vi "Version_2.0_Single_Column_Code.vi"() -> ()   [LabVIEW 2020] (continued)
                                n401 = local read "VISA Refnum in\nfor Pump"() -> (w876:refnum<visa-resource-name>)
                                n402 = local read "Port for \nA1-Equilibriation"() -> (w875:string)
                                n403 = call "PortChanger (SubVI).vi"("Port Number"=w875, "VISA Refnum in"=w876) -> ()  [unwired: 10 in]
                                }
                                frame #1 {
                                n404 = local read "VISA Refnum in\nfor Pump"() -> (w877:refnum<visa-resource-name>)
                                n405 = call "ProcessCompletionWaiter (SubVI).vi"("VISA Refnum in"=w877) -> ()  [unwired: 11 in]
                                }
                                frame #2 {
                                n406 = local read "VISA Refnum in\nfor Pump"() -> (w882:refnum<visa-resource-name>)
                                n407 = local read "Apparent Volume\nof Syringe"() -> (w878:dbl)
                                n408 = local read "Volume of Syringe"() -> (w879:dbl)
                                n409 = call "RPickUp(SubVI).vi"("Volume to be picked up"=w878, "Volume of Syringe"=w879, "Resolution of PickUP"=T2."Standard Pumping", "PickUp Flow Rate (ul/min)"=150.0, "VISA Refnum in"=w882) -> ()  [unwired: 6 in, 1 out]
                                }
                                frame #3 {
                                n410 = local read "Stopper that ends \nthe main loops"() -> (w883:bool)
                                n411 = local read "VISA Refnum in\nfor Pump"() -> (w884:refnum<visa-resource-name>)
                                n412 = case shown="True" w883 {
                                frame False {
                                }
                                frame True {
                                n413 = local read "VISA Refnum in\nfor Pump"() -> (w885:refnum<visa-resource-name>)
                                n414 = call "HardStopCurrentProcess (SubVI).vi"("VISA Refnum in"=w885) -> ()  [unwired: 11 in]
                                }
                                }
                                n415 = call "ProcessCompletionWaiter (SubVI).vi"("VISA Refnum in"=w884) -> ()  [unwired: 11 in]
                                }
                                frame #4 {
                                n416 = local read "VISA Refnum in\nfor Pump"() -> (w887:refnum<visa-resource-name>)
                                n417 = call "PortChanger (SubVI).vi"("Port Number"="1", "VISA Refnum in"=w887) -> ()  [unwired: 10 in]
                                }
                                frame #5 {
                                n418 = local read "Stopper that ends \nthe main loops"() -> (w888:bool)
                                n419 = local read "VISA Refnum in\nfor Pump"() -> (w889:refnum<visa-resource-name>)
                                n420 = case shown="True" w888 {
                                frame False {
                                }
                                frame True {
                                n421 = local read "VISA Refnum in\nfor Pump"() -> (w890:refnum<visa-resource-name>)
                                n422 = call "HardStopCurrentProcess (SubVI).vi"("VISA Refnum in"=w890) -> ()  [unwired: 11 in]
                                }
                                }
                                n423 = call "ProcessCompletionWaiter (SubVI).vi"("VISA Refnum in"=w889) -> ()  [unwired: 11 in]
                                }
                                frame #6 {
                                n424 = local read "VISA Refnum in\nfor Pump"() -> (w895:refnum<visa-resource-name>)
                                n425 = local read "Volume of Syringe"() -> (w892:dbl)
                                n426 = call "GoToAbsolutePosition(SubVI).vi"("Absolute Volume Position in Syringe (in ul)"=0.0 ("Volume to be picked up"), "Volume of Syringe"=w892, "Resolution of Pumping"=T2."Standard Pumping" ("Resolution of PickUP"), "Flow Rate (ul/min)"=150.0 ("PickUp Flow Rate (ul/min)"), "VISA Refnum in"=w895) -> ()  [unwired: 6 in, 1 out]
                                }
                                frame #7 {
                                n427 = local read "Stopper that ends \nthe main loops"() -> (w896:bool)
                                n428 = local read "VISA Refnum in\nfor Pump"() -> (w897:refnum<visa-resource-name>)
                                n429 = case shown="True" w896 {
                                frame False {
                                }
                                frame True {
                                n430 = local read "VISA Refnum in\nfor Pump"() -> (w898:refnum<visa-resource-name>)
                                n431 = call "HardStopCurrentProcess (SubVI).vi"("VISA Refnum in"=w898) -> ()  [unwired: 11 in]
                                }
                                }
                                n432 = call "ProcessCompletionWaiter (SubVI).vi"("VISA Refnum in"=w897) -> ()  [unwired: 11 in]
                                }
                              }
                              n433 = local write "Pause Data Collection"(TRUE ("Pause Data Collection")) -> ()
                            }
                          }
                          frame #2 {
                            # "Switch to Port-4"
                            # "Port-4 of pump is connected to Buffer-A1"
                            n434 = local read "Port for \nA1-Equilibriation"() -> (w899:string)
                            n435 = local read "VISA Refnum in\nfor Pump"() -> (w900:refnum<visa-resource-name>)
                            n436 = call "PortChanger (SubVI).vi"("Port Number"=w899, "VISA Refnum in"=w900) -> ()  [unwired: 10 in]
                          }
                          frame #3 {
                            n437 = local read "VISA Refnum in\nfor Pump"() -> (w901:refnum<visa-resource-name>)
                            n438 = call "ProcessCompletionWaiter (SubVI).vi"("VISA Refnum in"=w901) -> ()  [unwired: 11 in]
                          }
                          frame #4 {
                            n439 = local read "VISA Refnum in\nfor Valve"() -> (w908:refnum<visa-resource-name>)
                            n440 = local read "External Valve \nOPEN"() -> (w907:string)
                            n441 = local write "Valve V3 Open"(FALSE ("Valve V3 Open")) -> ()
                            n442 = local write "Valve V4 Open"(FALSE ("Valve V4 Open")) -> ()
                            n443 = local write "Valve V1 Open"(TRUE ("Valve V1 Open")) -> ()
                            n444 = local write "Valve V2 Open"(TRUE ("Valve V2 Open")) -> ()
                            n445 = call "PortChanger_Valve (SubVI).vi"("Port Number"=w907, "VISA Refnum in"=w908) -> ()  [unwired: 10 in]
                            n446 = local write "Valve V6 Open"(FALSE ("Valve V6 Open")) -> ()
                            n447 = local write "Valve V5 Open"(FALSE ("Valve V5 Open")) -> ()
                            n448 = local write "Valve V7 Open"(FALSE ("Valve V7 Open")) -> ()
                          }
                          frame #5 {
                            n449 = local read "Buffer-A1 Volume \nto be  Pumped \nfor Equilibration\nof Column-1"() -> (w914:dbl)
                            n450 = local read "Apparent Volume\nof Syringe"() -> (w911:dbl)
                            n451 = Quotient & Remainder(x=w914, y=w911) -> (x-y*floor(x/y)=w912:dbl, floor(x/y)=w913:dbl)
                            n452 = for {
                              N: w913 -> [_]
                              n453 = stacked-sequence {
                                frame #0 {
                                n454 = local read "Buffer-A1 PickUp \nFlow Rate (ul/min)\nfor Equilibration \nof Column-1"() -> (w917:dbl)
                                n455 = local read "Buffer-A1 Pumping\nResolution \nfor Equilibration \nof Column-1"() -> (w916:T2)
                                n456 = local read "VISA Refnum in\nfor Pump"() -> (w919:refnum<visa-resource-name>)
                                n457 = local read "Apparent Volume\nof Syringe"() -> (w915:dbl)
                                n458 = local read "Volume of Syringe"() -> (w918:dbl)
                                n459 = call "RPickUp(SubVI).vi"("Volume to be picked up"=w915, "Volume of Syringe"=w918, "Resolution of PickUP"=w916, "PickUp Flow Rate (ul/min)"=w917, "VISA Refnum in"=w919) -> ()  [unwired: 6 in, 1 out]
                                }
                                frame #1 {
                                n460 = while {
                                stop <- w920 stop-if-true
                                n461 = local read "Stopper that ends \nthe main loops"() -> (w921:bool)
                                n462 = local read "VISA Refnum in\nfor Pump"() -> (w922:refnum<visa-resource-name>)
                                n463 = case shown="True" w921 {
                                frame False {
                                }
                                frame True {
                                n464 = local read "VISA Refnum in\nfor Pump"() -> (w923:refnum<visa-resource-name>)
                                n465 = call "HardStopCurrentProcess (SubVI).vi"("VISA Refnum in"=w923) -> ()  [unwired: 11 in]
                                }
                                }
                                n466 = call "ProcessCompletionWaiterWithOutPut (SubVI).vi"("VISA Refnum in"=w922) -> ("Boolean"=w920:bool)  [unwired: 10 in]
                                }
                                }
                                frame #2 {
                                # "Reads the initial Plunger Position for computing the volume dispensed"
                                n467 = local read "VISA Refnum in\nfor Pump"() -> (w925:refnum<visa-resource-name>)
                                n468 = call "AbsolutePlungerPosition (SubVI).vi"("VISA Refnum in"=w925) -> ("Plunger Position"=w924:i32)  [unwired: 10 in]
                                n469 = local write "Initial Plunger Position"(w924) -> ()
                                }
                                frame #3 {
                                # "Switch to Port-2"
                                # "Port-2 of the pump is conncted to column-1 of chip"
                                n470 = local read "VISA Refnum in\nfor Pump"() -> (w927:refnum<visa-resource-name>)
                                n471 = call "PortChanger (SubVI).vi"("Port Number"="2", "VISA Refnum in"=w927) -> ()  [unwired: 10 in]
                                }
                                frame #4 {
                                n472 = while {
                                stop <- w928 stop-if-true
                                n473 = local read "Stopper that ends \nthe main loops"() -> (w929:bool)
                                n474 = local read "VISA Refnum in\nfor Pump"() -> (w930:refnum<visa-resource-name>)
                                n475 = case shown="True" w929 {
                                frame False {
                                }
                                frame True {
                                n476 = local read "VISA Refnum in\nfor Pump"() -> (w931:refnum<visa-resource-name>)
                                n477 = call "HardStopCurrentProcess (SubVI).vi"("VISA Refnum in"=w931) -> ()  [unwired: 11 in]
                                }
                                }
                                n478 = call "ProcessCompletionWaiterWithOutPut (SubVI).vi"("VISA Refnum in"=w930) -> ("Boolean"=w928:bool)  [unwired: 10 in]
                                }
                                }
                                frame #5 {
                                n479 = local read "Buffer-A1 Dispense\nFlow Rate (ul/min) \nfor Equilibration\nof Column-1"() -> (w935:dbl)
                                n480 = local read "Buffer-A1 Pumping\nResolution \nfor Equilibration \nof Column-1"() -> (w934:T2)
                                n481 = local read "VISA Refnum in\nfor Pump"() -> (w937:refnum<visa-resource-name>)
                                n482 = local write "Pause Data Collection"(FALSE ("Pause Data Collection")) -> ()
                                n483 = local read "Volume of Syringe"() -> (w936:dbl)
                                n484 = call "GoToAbsolutePosition(SubVI).vi"("Absolute Volume Position in Syringe (in ul)"=0.0, "Volume of Syringe"=w936, "Resolution of Pumping"=w934, "Flow Rate (ul/min)"=w935, "VISA Refnum in"=w937) -> ()  [unwired: 6 in, 1 out]
                                }
                                frame #6 {
                                n485 = local read "Buffer-A1 Pumping\nResolution \nfor Equilibration \nof Column-1"() -> (w939:T2)
                                n486 = local read "VISA Refnum in\nfor Pump"() -> (w941:refnum<visa-resource-name>)
                                n487 = local read "Initial Plunger Position"() -> (w940:dbl)
                                n488 = local read "Volume of Syringe"() -> (w938:dbl)
                                n489 = while {
                                tunnel: w940 -> [w948]
                                tunnel: w941 -> [w947]
                                tunnel: w939 -> [w946]
                                tunnel: w938 -> [w945]
                                stop <- w943 stop-if-true
                                n490 = stacked-sequence {
                                tunnel: w948 -> [w955 _]
                                tunnel: w947 -> [w954 w975]
                                tunnel: w946 -> [w953 _]
                                tunnel: w945 -> [w952 _]
                                tunnel: [_ w973] -> w943
                                frame #0 {
                                n491 = call "AbsolutePlungerPosition (SubVI).vi"("VISA Refnum in"=w954) -> ("Plunger Position"=w951:i32)  [unwired: 10 in]
                                n492 = case shown="\"Standard Pumping\", Default" w953 {
                                tunnel: w955 -> [w960 w969]
                                tunnel: w951 -> [w961 w968]
                                tunnel: [w959 w966] -> w950
                                tunnel: w952 -> [w958 w967]
                                frame "Standard Pumping", Default {
                                n493 = Subtract(x=w960, y=w961) -> (x-y=w957:dbl)
                                n494 = Absolute Value(x=w957) -> (abs(x)=w956:dbl)
                                n495 = Multiply(x=w956, y=w958) -> (x*y=w963:dbl)
                                n496 = Divide(x=w963, y=3000.0) -> (x/y=w959:dbl)
                                }
                                frame "High Resolution Pumping" {
                                n497 = Subtract(x=w969, y=w968) -> (x-y=w965:dbl)
                                n498 = Absolute Value(x=w965) -> (abs(x)=w964:dbl)
                                n499 = Multiply(x=w964, y=w967) -> (x*y=w971:dbl)
                                n500 = Divide(x=w971, y=24000.0) -> (x/y=w966:dbl)
                                }
                                }
                                n501 = local write "Volume being Injected \nin this process"(w950) -> ()
                                }
                                frame #1 {
                                n502 = call "LSPOneStatus (SubVI).vi"("VISA Refnum in"=w975) -> ("read buffer"=w977:string)  [unwired: 10 in]
                                n503 = call <vilib>:"Trim Whitespace.vi"("string"=w977) -> ("trimmed string"=w976:string)  [unwired: 1 in]
                                n504 = local read "Stopper that ends \nthe main loops"() -> (w972:bool)
                                n505 = Equal?(x=w976, y="/0`\u0003") -> (x = y?=w974:bool)
                                n506 = Or(x=w974, y=w972) -> (x .or. y?=w973:bool)
                                }
                                }
                                n507 = Wait (ms)(milliseconds to wait=u32 100) -> ()  [unwired: 1 out]
                                n508 = local read "Stopper that ends \nthe main loops"() -> (w942:bool)
                                n509 = case shown="True" w942 {
                                frame False {
                                }
                                frame True {
                                n510 = local read "VISA Refnum in\nfor Pump"() -> (w949:refnum<visa-resource-name>)
                                n511 = call "HardStopCurrentProcess (SubVI).vi"("VISA Refnum in"=w949) -> ()  [unwired: 11 in]
                                }
                                }
                                }
                                }
                                frame #7 {
                                # "Change the pump port back to Buffer-A1"
                                n512 = local read "VISA Refnum in\nfor Pump"() -> (w980:refnum<visa-resource-name>)
                                n513 = local read "Port for \nA1-Equilibriation"() -> (w979:string)
                                n514 = local write "Pause Data Collection"(TRUE ("Pause Data Collection")) -> ()
                                n515 = Wait (ms)(milliseconds to wait=u32 500) -> ()  [unwired: 1 out]
                                n516 = call "PortChanger (SubVI).vi"("Port Number"=w979, "VISA Refnum in"=w980) -> ()  [unwired: 10 in]
                                }
                                frame #8 {
                                n517 = local read "VISA Refnum in\nfor Pump"() -> (w983:refnum<visa-resource-name>)
                                n518 = local write "Volume being Injected \nin this process"(0.0 ("Volume being Injected \nin this process")) -> ()
                                n519 = call "ProcessCompletionWaiter (SubVI).vi"("VISA Refnum in"=w983) -> ()  [unwired: 11 in]
                                }
                              }
                            }
                            n520 = local write "Reminder of the \nVolume to be \nPumped"(w912) -> ()
                          }
                          frame #6 {
                            n521 = stacked-sequence {
                              frame #0 {
                                n522 = local read "Buffer-A1 PickUp \nFlow Rate (ul/min)\nfor Equilibration \nof Column-1"() -> (w987:dbl)
                                n523 = local read "Buffer-A1 Pumping\nResolution \nfor Equilibration \nof Column-1"() -> (w986:T2)
                                n524 = local read "VISA Refnum in\nfor Pump"() -> (w989:refnum<visa-resource-name>)
                                n525 = local read "Reminder of the \nVolume to be \nPumped"() -> (w985:dbl)
                                n526 = local read "Volume of Syringe"() -> (w988:dbl)
                                n527 = call "RPickUp(SubVI).vi"("Volume to be picked up"=w985, "Volume of Syringe"=w988, "Resolution of PickUP"=w986, "PickUp Flow Rate (ul/min)"=w987, "VISA Refnum in"=w989) -> ()  [unwired: 6 in, 1 out]
                              }
                              frame #1 {
                                n528 = while {
                                stop <- w990 stop-if-true
                                n529 = local read "Stopper that ends \nthe main loops"() -> (w991:bool)
                                n530 = local read "VISA Refnum in\nfor Pump"() -> (w992:refnum<visa-resource-name>)
                                n531 = case shown="True" w991 {
                                frame False {
                                }
                                frame True {
                                n532 = local read "VISA Refnum in\nfor Pump"() -> (w993:refnum<visa-resource-name>)
                                n533 = call "HardStopCurrentProcess (SubVI).vi"("VISA Refnum in"=w993) -> ()  [unwired: 11 in]
                                }
                                }
                                n534 = call "ProcessCompletionWaiterWithOutPut (SubVI).vi"("VISA Refnum in"=w992) -> ("Boolean"=w990:bool)  [unwired: 10 in]
                                }
                              }
                              frame #2 {
                                # "Reads the initial Plunger Position for computing the volume dispensed"
                                n535 = local read "VISA Refnum in\nfor Pump"() -> (w995:refnum<visa-resource-name>)
                                n536 = call "AbsolutePlungerPosition (SubVI).vi"("VISA Refnum in"=w995) -> ("Plunger Position"=w994:i32)  [unwired: 10 in]
                                n537 = local write "Initial Plunger Position"(w994) -> ()
                              }
                              frame #3 {
                                # "Switch to Port-2"
                                # "Port-2 of the pump is conncted to column-1 of chip"
                                n538 = local read "VISA Refnum in\nfor Pump"() -> (w997:refnum<visa-resource-name>)
                                n539 = call "PortChanger (SubVI).vi"("Port Number"="2", "VISA Refnum in"=w997) -> ()  [unwired: 10 in]
                              }
                              frame #4 {
                                n540 = while {
                                stop <- w998 stop-if-true
                                n541 = local read "Stopper that ends \nthe main loops"() -> (w999:bool)
                                n542 = local read "VISA Refnum in\nfor Pump"() -> (w1000:refnum<visa-resource-name>)
                                n543 = case shown="True" w999 {
                                frame False {
                                }
                                frame True {
                                n544 = local read "VISA Refnum in\nfor Pump"() -> (w1001:refnum<visa-resource-name>)
                                n545 = call "HardStopCurrentProcess (SubVI).vi"("VISA Refnum in"=w1001) -> ()  [unwired: 11 in]
                                }
                                }
                                n546 = call "ProcessCompletionWaiterWithOutPut (SubVI).vi"("VISA Refnum in"=w1000) -> ("Boolean"=w998:bool)  [unwired: 10 in]
                                }
                              }
                              frame #5 {
                                n547 = local read "Buffer-A1 Pumping\nResolution \nfor Equilibration \nof Column-1"() -> (w1004:T2)
                                n548 = local read "Buffer-A1 Dispense\nFlow Rate (ul/min) \nfor Equilibration\nof Column-1"() -> (w1005:dbl)
                                n549 = local read "VISA Refnum in\nfor Pump"() -> (w1007:refnum<visa-resource-name>)
                                n550 = local write "Pause Data Collection"(FALSE ("Pause Data Collection")) -> ()
                                n551 = local read "Volume of Syringe"() -> (w1006:dbl)
                                n552 = call "GoToAbsolutePosition(SubVI).vi"("Absolute Volume Position in Syringe (in ul)"=0.0 ("Volume to be Dispensed"), "Volume of Syringe"=w1006, "Resolution of Pumping"=w1004, "Flow Rate (ul/min)"=w1005, "VISA Refnum in"=w1007) -> ()  [unwired: 6 in, 1 out]
                              }
                              frame #6 {
                                n553 = local read "Buffer-A1 Pumping\nResolution \nfor Equilibration \nof Column-1"() -> (w1009:T2)
                                n554 = local read "VISA Refnum in\nfor Pump"() -> (w1011:refnum<visa-resource-name>)
                                n555 = local read "Initial Plunger Position"() -> (w1010:dbl)
                                n556 = local read "Volume of Syringe"() -> (w1008:dbl)
                                n557 = while {
                                tunnel: w1010 -> [w1018]
                                tunnel: w1011 -> [w1017]
                                tunnel: w1009 -> [w1016]
                                tunnel: w1008 -> [w1015]
                                stop <- w1013 stop-if-true
                                n558 = stacked-sequence {
                                tunnel: w1018 -> [w1025 _]
                                tunnel: w1017 -> [w1024 w1045]
                                tunnel: w1016 -> [w1023 _]
                                tunnel: w1015 -> [w1022 _]
                                tunnel: [_ w1043] -> w1013
                                frame #0 {
                                n559 = call "AbsolutePlungerPosition (SubVI).vi"("VISA Refnum in"=w1024) -> ("Plunger Position"=w1021:i32)  [unwired: 10 in]
                                n560 = case shown="\"Standard Pumping\", Default" w1023 {
                                tunnel: w1025 -> [w1030 w1039]
                                tunnel: w1021 -> [w1031 w1038]
                                tunnel: [w1029 w1036] -> w1020
                                tunnel: w1022 -> [w1028 w1037]
                                frame "Standard Pumping", Default {
                                n561 = Subtract(x=w1030, y=w1031) -> (x-y=w1027:dbl)
                                n562 = Absolute Value(x=w1027) -> (abs(x)=w1026:dbl)
                                n563 = Multiply(x=w1026, y=w1028) -> (x*y=w1033:dbl)
                                n564 = Divide(x=w1033, y=3000.0) -> (x/y=w1029:dbl)
                                }
                                frame "High Resolution Pumping" {
                                n565 = Subtract(x=w1039, y=w1038) -> (x-y=w1035:dbl)
                                n566 = Absolute Value(x=w1035) -> (abs(x)=w1034:dbl)
                                n567 = Multiply(x=w1034, y=w1037) -> (x*y=w1041:dbl)
                                n568 = Divide(x=w1041, y=24000.0) -> (x/y=w1036:dbl)
                                }
                                }
                                n569 = local write "Volume being Injected \nin this process"(w1020) -> ()
                                }
                                frame #1 {
                                n570 = call "LSPOneStatus (SubVI).vi"("VISA Refnum in"=w1045) -> ("read buffer"=w1047:string)  [unwired: 10 in]
                                n571 = call <vilib>:"Trim Whitespace.vi"("string"=w1047) -> ("trimmed string"=w1046:string)  [unwired: 1 in]
                                n572 = local read "Stopper that ends \nthe main loops"() -> (w1042:bool)
                                n573 = Equal?(x=w1046, y="/0`\u0003") -> (x = y?=w1044:bool)
                                n574 = Or(x=w1044, y=w1042) -> (x .or. y?=w1043:bool)
                                }
                                }
                                n575 = Wait (ms)(milliseconds to wait=u32 100) -> ()  [unwired: 1 out]
                                n576 = local read "Stopper that ends \nthe main loops"() -> (w1012:bool)
                                n577 = case shown="True" w1012 {
                                frame False {
                                }
                                frame True {
                                n578 = local read "VISA Refnum in\nfor Pump"() -> (w1019:refnum<visa-resource-name>)
                                n579 = call "HardStopCurrentProcess (SubVI).vi"("VISA Refnum in"=w1019) -> ()  [unwired: 11 in]
                                }
                                }
                                }
                              }
                              frame #7 {
                                # "Change the pump port to Buffer-C1 for equilibriation of column-2"
                                n580 = local read "VISA Refnum in\nfor Pump"() -> (w1050:refnum<visa-resource-name>)
                                n581 = local read "Port for \nC1-Equilibriation"() -> (w1049:string)
                                n582 = local write "Pause Data Collection"(TRUE ("Pause Data Collection")) -> ()
                                n583 = Wait (ms)(milliseconds to wait=u32 500) -> ()  [unwired: 1 out]
                                n584 = call "PortChanger (SubVI).vi"("Port Number"=w1049, "VISA Refnum in"=w1050) -> ()  [unwired: 10 in]
                              }
                              frame #8 {
                                n585 = local read "VISA Refnum in\nfor Pump"() -> (w1054:refnum<visa-resource-name>)
                                n586 = local write "Volume being Injected \nin this process"(0.0 ("Volume being Injected \nin this process")) -> ()
                                n587 = call "ProcessCompletionWaiter (SubVI).vi"("VISA Refnum in"=w1054) -> ()  [unwired: 11 in]
                                n588 = local write "Start the Process"(FALSE ("Start the Process")) -> ()
                              }
                            }
                          }
                          frame #7 {
                            # "Clean the tubing with Buffer-C1"
                            n589 = local read "N-C1"() -> (w1057:i32)
                            n590 = local write "Equilibriating \nColumn-1"(FALSE ("Equilibriating \nColumn-1")) -> ()
                            n591 = for {
                              N: w1057 -> [_]
                              n592 = stacked-sequence {
                                frame #0 {
                                n593 = local read "Port for \nC1-Equilibriation"() -> (w1060:string)
                                n594 = local read "VISA Refnum in\nfor Pump"() -> (w1061:refnum<visa-resource-name>)
                                n595 = call "PortChanger (SubVI).vi"("Port Number"=w1060, "VISA Refnum in"=w1061) -> ()  [unwired: 10 in]
                                }
                                frame #1 {
                                n596 = local read "VISA Refnum in\nfor Pump"() -> (w1062:refnum<visa-resource-name>)
                                n597 = call "ProcessCompletionWaiter (SubVI).vi"("VISA Refnum in"=w1062) -> ()  [unwired: 11 in]
                                }
                                frame #2 {
                                n598 = local read "VISA Refnum in\nfor Pump"() -> (w1067:refnum<visa-resource-name>)
                                n599 = local read "Apparent Volume\nof Syringe"() -> (w1063:dbl)
                                n600 = local read "Volume of Syringe"() -> (w1064:dbl)
                                n601 = call "RPickUp(SubVI).vi"("Volume to be picked up"=w1063, "Volume of Syringe"=w1064, "Resolution of PickUP"=T2."Standard Pumping", "PickUp Flow Rate (ul/min)"=150.0, "VISA Refnum in"=w1067) -> ()  [unwired: 6 in, 1 out]
                                }
                                frame #3 {
                                n602 = local read "Stopper that ends \nthe main loops"() -> (w1068:bool)
                                n603 = local read "VISA Refnum in\nfor Pump"() -> (w1069:refnum<visa-resource-name>)
                                n604 = case shown="True" w1068 {
                                frame False {
                                }
                                frame True {
                                n605 = local read "VISA Refnum in\nfor Pump"() -> (w1070:refnum<visa-resource-name>)
                                n606 = call "HardStopCurrentProcess (SubVI).vi"("VISA Refnum in"=w1070) -> ()  [unwired: 11 in]
                                }
                                }
                                n607 = call "ProcessCompletionWaiter (SubVI).vi"("VISA Refnum in"=w1069) -> ()  [unwired: 11 in]
                                }
                                frame #4 {
                                n608 = local read "VISA Refnum in\nfor Pump"() -> (w1072:refnum<visa-resource-name>)
                                n609 = call "PortChanger (SubVI).vi"("Port Number"="1", "VISA Refnum in"=w1072) -> ()  [unwired: 10 in]
                                }
                                frame #5 {
                                n610 = local read "Stopper that ends \nthe main loops"() -> (w1073:bool)
                                n611 = local read "VISA Refnum in\nfor Pump"() -> (w1074:refnum<visa-resource-name>)
                                n612 = case shown="True" w1073 {
                                frame False {
                                }
                                frame True {
                                n613 = local read "VISA Refnum in\nfor Pump"() -> (w1075:refnum<visa-resource-name>)
                                n614 = call "HardStopCurrentProcess (SubVI).vi"("VISA Refnum in"=w1075) -> ()  [unwired: 11 in]
                                }
                                }
                                n615 = call "ProcessCompletionWaiter (SubVI).vi"("VISA Refnum in"=w1074) -> ()  [unwired: 11 in]
                                }
                                frame #6 {
                                n616 = local read "VISA Refnum in\nfor Pump"() -> (w1080:refnum<visa-resource-name>)
                                n617 = local read "Volume of Syringe"() -> (w1077:dbl)
                                n618 = call "GoToAbsolutePosition(SubVI).vi"("Absolute Volume Position in Syringe (in ul)"=0.0 ("Volume to be picked up"), "Volume of Syringe"=w1077, "Resolution of Pumping"=T2."Standard Pumping" ("Resolution of PickUP"), "Flow Rate (ul/min)"=150.0 ("PickUp Flow Rate (ul/min)"), "VISA Refnum in"=w1080) -> ()  [unwired: 6 in, 1 out]
                                }
                                frame #7 {
                                n619 = local read "Stopper that ends \nthe main loops"() -> (w1081:bool)
                                n620 = local read "VISA Refnum in\nfor Pump"() -> (w1082:refnum<visa-resource-name>)
                                n621 = case shown="True" w1081 {
                                frame False {
                                }
                                frame True {
                                n622 = local read "VISA Refnum in\nfor Pump"() -> (w1083:refnum<visa-resource-name>)
                                n623 = call "HardStopCurrentProcess (SubVI).vi"("VISA Refnum in"=w1083) -> ()  [unwired: 11 in]
                                }
                                }
                                n624 = call "ProcessCompletionWaiter (SubVI).vi"("VISA Refnum in"=w1082) -> ()  [unwired: 11 in]
                                }
                              }
                            }
                            n625 = local write "Pause Data Collection"(TRUE ("Pause Data Collection")) -> ()
                            n626 = local write "Equilibriating \nColumn-2"(TRUE ("Equilibriating \nColumn-2")) -> ()
                          }
                          frame #8 {
                            n627 = local read "Buffer-C1 Volume \nto be  Pumped \nfor Equilibration\nof Column-2"() -> (w1087:dbl)
                            n628 = local read "Apparent Volume\nof Syringe"() -> (w1084:dbl)
                            n629 = Quotient & Remainder(x=w1087, y=w1084) -> (x-y*floor(x/y)=w1085:dbl, floor(x/y)=w1086:dbl)
                            n630 = for {
                              N: w1086 -> [_]
                              n631 = stacked-sequence {
                                frame #0 {
                                n632 = local read "VISA Refnum in\nfor Pump"() -> (w1089:refnum<visa-resource-name>)
                                n633 = local read "Port for \nC1-Equilibriation"() -> (w1088:string)
                                n634 = call "PortChanger (SubVI).vi"("Port Number"=w1088, "VISA Refnum in"=w1089) -> ()  [unwired: 10 in]
                                }
                                frame #1 {
                                n635 = local read "VISA Refnum in\nfor Pump"() -> (w1090:refnum<visa-resource-name>)
                                n636 = call "ProcessCompletionWaiter (SubVI).vi"("VISA Refnum in"=w1090) -> ()  [unwired: 11 in]
                                }
                                frame #2 {
                                n637 = local read "Buffer-C1 PickUp \nFlow Rate (ul/min)\nfor Equilibration \nof Column-2"() -> (w1093:dbl)
                                n638 = local read "Buffer-C1 Pumping\nResolution \nfor Equilibration \nof Column-2"() -> (w1092:T2)
                                n639 = local read "VISA Refnum in\nfor Pump"() -> (w1095:refnum<visa-resource-name>)
                                n640 = local read "Apparent Volume\nof Syringe"() -> (w1091:dbl)
                                n641 = local read "Volume of Syringe"() -> (w1094:dbl)
                                n642 = call "RPickUp(SubVI).vi"("Volume to be picked up"=w1091, "Volume of Syringe"=w1094, "Resolution of PickUP"=w1092, "PickUp Flow Rate (ul/min)"=w1093, "VISA Refnum in"=w1095) -> ()  [unwired: 6 in, 1 out]
                                }
                                frame #3 {
                                n643 = while {
                                stop <- w1096 stop-if-true
                                n644 = local read "Stopper that ends \nthe main loops"() -> (w1097:bool)
                                n645 = local read "VISA Refnum in\nfor Pump"() -> (w1098:refnum<visa-resource-name>)
                                n646 = case shown="True" w1097 {
                                frame False {
                                }
                                frame True {
                                n647 = local read "VISA Refnum in\nfor Pump"() -> (w1099:refnum<visa-resource-name>)
                                n648 = call "HardStopCurrentProcess (SubVI).vi"("VISA Refnum in"=w1099) -> ()  [unwired: 11 in]
                                }
                                }
                                n649 = call "ProcessCompletionWaiterWithOutPut (SubVI).vi"("VISA Refnum in"=w1098) -> ("Boolean"=w1096:bool)  [unwired: 10 in]
                                }
                                }
                                frame #4 {
                                # "Reads the initial Plunger Position for computing the volume dispensed"
                                n650 = local read "VISA Refnum in\nfor Pump"() -> (w1101:refnum<visa-resource-name>)
                                n651 = call "AbsolutePlungerPosition (SubVI).vi"("VISA Refnum in"=w1101) -> ("Plunger Position"=w1100:i32)  [unwired: 10 in]
                                n652 = local write "Initial Plunger Position"(w1100) -> ()
                                }
                                frame #5 {
                                # "Switch to Port-10"
                                # "Port-10 of the pump is conncted to column-2 of chip"
                                n653 = local read "VISA Refnum in\nfor Pump"() -> (w1103:refnum<visa-resource-name>)
                                n654 = call "PortChanger (SubVI).vi"("Port Number"="10", "VISA Refnum in"=w1103) -> ()  [unwired: 10 in]
                                }
                                frame #6 {
                                n655 = while {
                                stop <- w1104 stop-if-true
                                n656 = local read "Stopper that ends \nthe main loops"() -> (w1105:bool)
                                n657 = local read "VISA Refnum in\nfor Pump"() -> (w1106:refnum<visa-resource-name>)
                                n658 = case shown="True" w1105 {
                                frame False {
                                }
                                frame True {
                                n659 = local read "VISA Refnum in\nfor Pump"() -> (w1107:refnum<visa-resource-name>)
                                n660 = call "HardStopCurrentProcess (SubVI).vi"("VISA Refnum in"=w1107) -> ()  [unwired: 11 in]
                                }
                                }
                                n661 = call "ProcessCompletionWaiterWithOutPut (SubVI).vi"("VISA Refnum in"=w1106) -> ("Boolean"=w1104:bool)  [unwired: 10 in]
                                }
                                }
                                frame #7 {
                                # "Buffer-C pumped for column non-interference"
                                # "Keeps the AMF valve after column-1 open and valve after column-2 closed"
                                n662 = local read "Buffer-C1 Dispense\nFlow Rate (ul/min) \nfor Equilibration\nof Column-2"() -> (w1120:dbl)
                                n663 = local read "Buffer-C1 Pumping\nResolution \nfor Equilibration \nof Column-2"() -> (w1119:T2)
                                n664 = local read "VISA Refnum in\nfor Pump"() -> (w1122:refnum<visa-resource-name>)
                                n665 = local write "Pause Data Collection"(FALSE ("Pause Data Collection")) -> ()
                                n666 = local read "Volume of Syringe"() -> (w1121:dbl)
                                n667 = call "GoToAbsolutePosition(SubVI).vi"("Absolute Volume Position in Syringe (in ul)"=0.0, "Volume of Syringe"=w1121, "Resolution of Pumping"=w1119, "Flow Rate (ul/min)"=w1120, "VISA Refnum in"=w1122) -> ()  [unwired: 6 in, 1 out]
                                n668 = local write "Valve V1 Open"(FALSE ("Valve V1 Open")) -> ()
                                n669 = local write "Valve V2 Open"(TRUE ("Valve V2 Open")) -> ()
                                n670 = local write "Valve V4 Open"(FALSE ("Valve V4 Open")) -> ()
                                n671 = local write "Valve V3 Open"(TRUE ("Valve V3 Open")) -> ()
                                n672 = local read "VISA Refnum in\nfor Valve"() -> (w1113:refnum<visa-resource-name>)
                                n673 = local read "External Valve \nOPEN"() -> (w1112:string)
                                n674 = local write "Valve V5 Open"(FALSE ("Valve V5 Open")) -> ()
                                n675 = local write "Valve V6 Open"(FALSE ("Valve V6 Open")) -> ()
                                n676 = local write "Valve V7 Open"(FALSE ("Valve V7 Open")) -> ()
                                n677 = call "PortChanger_Valve (SubVI).vi"("Port Number"=w1112, "VISA Refnum in"=w1113) -> ()  [unwired: 10 in]
                                }
                                frame #8 {
                                n678 = local read "Buffer-C1 Pumping\nResolution \nfor Equilibration \nof Column-2"() -> (w1124:T2)
                                n679 = local read "VISA Refnum in\nfor Pump"() -> (w1126:refnum<visa-resource-name>)
                                n680 = local read "Initial Plunger Position"() -> (w1125:dbl)
                                n681 = local read "Volume of Syringe"() -> (w1123:dbl)
                                n682 = while {
                                tunnel: w1125 -> [w1133]
                                tunnel: w1126 -> [w1132]
                                tunnel: w1124 -> [w1131]
                                tunnel: w1123 -> [w1130]
                                stop <- w1128 stop-if-true
                                n683 = stacked-sequence {
                                tunnel: w1133 -> [w1140 _]
                                tunnel: w1132 -> [w1139 w1164]
                                tunnel: w1131 -> [w1138 _]
                                tunnel: w1130 -> [w1137 _]
                                tunnel: [_ w1162] -> w1128
                                frame #0 {
                                n684 = call "AbsolutePlungerPosition (SubVI).vi"("VISA Refnum in"=w1139) -> ("Plunger Position"=w1136:i32)  [unwired: 10 in]
                                n685 = case shown="\"Standard Pumping\", Default" w1138 {
                                tunnel: w1140 -> [w1145 w1154]
                                tunnel: w1136 -> [w1146 w1153]
                                tunnel: [w1144 w1151] -> w1135
                                tunnel: w1137 -> [w1143 w1152]
                                frame "Standard Pumping", Default {
                                n686 = Subtract(x=w1145, y=w1146) -> (x-y=w1142:dbl)
                                n687 = Absolute Value(x=w1142) -> (abs(x)=w1141:dbl)
                                n688 = Multiply(x=w1141, y=w1143) -> (x*y=w1148:dbl)
                                n689 = Divide(x=w1148, y=3000.0) -> (x/y=w1144:dbl)
                                }
                                frame "High Resolution Pumping" {
                                n690 = Subtract(x=w1154, y=w1153) -> (x-y=w1150:dbl)
                                n691 = Absolute Value(x=w1150) -> (abs(x)=w1149:dbl)
                                n692 = Multiply(x=w1149, y=w1152) -> (x*y=w1156:dbl)
                                n693 = Divide(x=w1156, y=24000.0) -> (x/y=w1151:dbl)
                                }
                                }
                                n694 = local write "Volume being Injected \nin this process"(w1135) -> ()
                                }
                                frame #1 {
                                n695 = local read "Buffer-C Volume \nto be Pumped for\nColumn \nnon-interference"() -> (w1160:dbl)
                                n696 = local read "Volume being Injected \nin this process"() -> (w1161:dbl)
                                n697 = local read "Stopper that ends \nthe main loops"() -> (w1159:bool)
                                n698 = call "LSPOneStatus (SubVI).vi"("VISA Refnum in"=w1164) -> ("read buffer"=w1166:string)  [unwired: 10 in]
                                n699 = call <vilib>:"Trim Whitespace.vi"("string"=w1166) -> ("trimmed string"=w1165:string)  [unwired: 1 in]
                                n700 = Equal?(x=w1165, y="/0`\u0003") -> (x = y?=w1163:bool)
                                n701 = Greater Or Equal?(x=w1161, y=w1160) -> (x >= y?=w1158:bool)
                                n702 = Or(x=w1159, y=w1158) -> (x .or. y?=w1157:bool)
                                n703 = Or(x=w1163, y=w1157) -> (x .or. y?=w1162:bool)
                                }
                                }
                                n704 = Wait (ms)(milliseconds to wait=u32 100) -> ()  [unwired: 1 out]
                                n705 = local read "Stopper that ends \nthe main loops"() -> (w1127:bool)
                                n706 = case shown="True" w1127 {
                                frame False {
                                }
                                frame True {
                                n707 = local read "VISA Refnum in\nfor Pump"() -> (w1134:refnum<visa-resource-name>)
                                n708 = call "HardStopCurrentProcess (SubVI).vi"("VISA Refnum in"=w1134) -> ()  [unwired: 11 in]
                                }
                                }
                                }
                                }
                                frame #9 {
                                # "Keeps the AMF valve after column-1 closed and valve after column-2 open"
                                n709 = local read "VISA Refnum in\nfor Valve"() -> (w1172:refnum<visa-resource-name>)
                                n710 = local read "External Valve \nCLOSED"() -> (w1171:string)
                                n711 = local write "Valve V3 Open"(FALSE ("Valve V3 Open")) -> ()
                                n712 = local write "Valve V2 Open"(FALSE ("Valve V2 Open")) -> ()
                                n713 = local write "Valve V4 Open"(TRUE ("Valve V1 Open")) -> ()
                                n714 = local write "Valve V1 Open"(FALSE ("Valve V1 Open")) -> ()
                                n715 = call "PortChanger_Valve (SubVI).vi"("Port Number"=w1171, "VISA Refnum in"=w1172) -> ()  [unwired: 10 in]
                                n716 = local write "Valve V5 Open"(TRUE ("Valve V4 Open")) -> ()
                                n717 = local write "Valve V7 Open"(TRUE ("Valve V6 Open")) -> ()
                                n718 = local write "Valve V6 Open"(FALSE ("Valve V6 Open")) -> ()
                                }
                                frame #10 {
                                n719 = local read "Buffer-C1 Pumping\nResolution \nfor Equilibration \nof Column-2"() -> (w1178:T2)
                                n720 = local read "VISA Refnum in\nfor Pump"() -> (w1180:refnum<visa-resource-name>)
                                n721 = local read "Initial Plunger Position"() -> (w1179:dbl)
                                n722 = local read "Volume of Syringe"() -> (w1177:dbl)
                                n723 = while {
                                tunnel: w1179 -> [w1187]
                                tunnel: w1180 -> [w1186]
                                tunnel: w1178 -> [w1185]
                                tunnel: w1177 -> [w1184]
                                stop <- w1182 stop-if-true
                                n724 = stacked-sequence {
                                tunnel: w1187 -> [w1194 _]
                                tunnel: w1186 -> [w1193 w1214]
                                tunnel: w1185 -> [w1192 _]
                                tunnel: w1184 -> [w1191 _]
                                tunnel: [_ w1212] -> w1182
                                frame #0 {
                                n725 = call "AbsolutePlungerPosition (SubVI).vi"("VISA Refnum in"=w1193) -> ("Plunger Position"=w1190:i32)  [unwired: 10 in]
                                n726 = case shown="\"Standard Pumping\", Default" w1192 {
                                tunnel: w1194 -> [w1199 w1208]
                                tunnel: w1190 -> [w1200 w1207]
                                tunnel: [w1198 w1205] -> w1189
                                tunnel: w1191 -> [w1197 w1206]
                                frame "Standard Pumping", Default {
                                n727 = Subtract(x=w1199, y=w1200) -> (x-y=w1196:dbl)
                                n728 = Absolute Value(x=w1196) -> (abs(x)=w1195:dbl)
                                n729 = Multiply(x=w1195, y=w1197) -> (x*y=w1202:dbl)
                                n730 = Divide(x=w1202, y=3000.0) -> (x/y=w1198:dbl)
                                }
                                frame "High Resolution Pumping" {
                                n731 = Subtract(x=w1208, y=w1207) -> (x-y=w1204:dbl)
                                n732 = Absolute Value(x=w1204) -> (abs(x)=w1203:dbl)
                                n733 = Multiply(x=w1203, y=w1206) -> (x*y=w1210:dbl)
                                n734 = Divide(x=w1210, y=24000.0) -> (x/y=w1205:dbl)
                                }
                                }
                                n735 = local write "Volume being Injected \nin this process"(w1189) -> ()
                                }
                                frame #1 {
                                n736 = local read "Stopper that ends \nthe main loops"() -> (w1211:bool)
                                n737 = call "LSPOneStatus (SubVI).vi"("VISA Refnum in"=w1214) -> ("read buffer"=w1216:string)  [unwired: 10 in]
                                n738 = call <vilib>:"Trim Whitespace.vi"("string"=w1216) -> ("trimmed string"=w1215:string)  [unwired: 1 in]
                                n739 = Equal?(x=w1215, y="/0`\u0003") -> (x = y?=w1213:bool)
                                n740 = Or(x=w1213, y=w1211) -> (x .or. y?=w1212:bool)
                                }
                                }
                                n741 = Wait (ms)(milliseconds to wait=u32 100) -> ()  [unwired: 1 out]
                                n742 = local read "Stopper that ends \nthe main loops"() -> (w1181:bool)
                                n743 = case shown="True" w1181 {
                                frame False {
                                }
                                frame True {
                                n744 = local read "VISA Refnum in\nfor Pump"() -> (w1188:refnum<visa-resource-name>)
                                n745 = call "HardStopCurrentProcess (SubVI).vi"("VISA Refnum in"=w1188) -> ()  [unwired: 11 in]
                                }
                                }
                                }
                                }
                                frame #11 {
                                # "Change the pump port back to Buffer-C1"
                                n746 = local read "VISA Refnum in\nfor Pump"() -> (w1219:refnum<visa-resource-name>)
                                n747 = local read "Port for \nC1-Equilibriation"() -> (w1218:string)
                                n748 = local write "Pause Data Collection"(TRUE ("Pause Data Collection")) -> ()
                                n749 = Wait (ms)(milliseconds to wait=u32 500) -> ()  [unwired: 1 out]
                                n750 = call "PortChanger (SubVI).vi"("Port Number"=w1218, "VISA Refnum in"=w1219) -> ()  [unwired: 10 in]
                                }
                                frame #12 {
                                n751 = local read "VISA Refnum in\nfor Pump"() -> (w1222:refnum<visa-resource-name>)
                                n752 = local write "Volume being Injected \nin this process"(0.0 ("Volume being Injected \nin this process")) -> ()
                                n753 = call "ProcessCompletionWaiter (SubVI).vi"("VISA Refnum in"=w1222) -> ()  [unwired: 11 in]
                                }
                              }
                            }
                            n754 = local write "Reminder of the \nVolume to be \nPumped"(w1085) -> ()
                          }
                          frame #9 {
                            n755 = stacked-sequence {
                              frame #0 {
                                n756 = local read "Buffer-C1 PickUp \nFlow Rate (ul/min)\nfor Equilibration \nof Column-2"() -> (w1226:dbl)
                                n757 = local read "Buffer-C1 Pumping\nResolution \nfor Equilibration \nof Column-2"() -> (w1225:T2)
                                n758 = local read "VISA Refnum in\nfor Pump"() -> (w1228:refnum<visa-resource-name>)
                                n759 = local read "Reminder of the \nVolume to be \nPumped"() -> (w1224:dbl)
                                n760 = local read "Volume of Syringe"() -> (w1227:dbl)
                                n761 = call "RPickUp(SubVI).vi"("Volume to be picked up"=w1224, "Volume of Syringe"=w1227, "Resolution of PickUP"=w1225, "PickUp Flow Rate (ul/min)"=w1226, "VISA Refnum in"=w1228) -> ()  [unwired: 6 in, 1 out]
                              }
                              frame #1 {
                                n762 = while {
                                stop <- w1229 stop-if-true
                                n763 = local read "Stopper that ends \nthe main loops"() -> (w1230:bool)
                                n764 = local read "VISA Refnum in\nfor Pump"() -> (w1231:refnum<visa-resource-name>)
                                n765 = case shown="True" w1230 {
                                frame False {
                                }
                                frame True {
                                n766 = local read "VISA Refnum in\nfor Pump"() -> (w1232:refnum<visa-resource-name>)
                                n767 = call "HardStopCurrentProcess (SubVI).vi"("VISA Refnum in"=w1232) -> ()  [unwired: 11 in]
                                }
                                }
                                n768 = call "ProcessCompletionWaiterWithOutPut (SubVI).vi"("VISA Refnum in"=w1231) -> ("Boolean"=w1229:bool)  [unwired: 10 in]
                                }
                              }
                              frame #2 {
                                # "Reads the initial Plunger Position for computing the volume dispensed"
                                n769 = local read "VISA Refnum in\nfor Pump"() -> (w1234:refnum<visa-resource-name>)
                                n770 = call "AbsolutePlungerPosition (SubVI).vi"("VISA Refnum in"=w1234) -> ("Plunger Position"=w1233:i32)  [unwired: 10 in]
                                n771 = local write "Initial Plunger Position"(w1233) -> ()
                              }
                              frame #3 {
                                # "Switch to Port-10"
                                # "Port-10 of the pump is conncted to column-2 of chip"
                                n772 = local read "VISA Refnum in\nfor Pump"() -> (w1236:refnum<visa-resource-name>)
                                n773 = call "PortChanger (SubVI).vi"("Port Number"="10", "VISA Refnum in"=w1236) -> ()  [unwired: 10 in]
                              }
                              frame #4 {
                                n774 = while {
                                stop <- w1237 stop-if-true
                                n775 = local read "Stopper that ends \nthe main loops"() -> (w1238:bool)
                                n776 = local read "VISA Refnum in\nfor Pump"() -> (w1239:refnum<visa-resource-name>)
                                n777 = case shown="True" w1238 {
                                frame False {
                                }
                                frame True {
                                n778 = local read "VISA Refnum in\nfor Pump"() -> (w1240:refnum<visa-resource-name>)
                                n779 = call "HardStopCurrentProcess (SubVI).vi"("VISA Refnum in"=w1240) -> ()  [unwired: 11 in]
                                }
                                }
                                n780 = call "ProcessCompletionWaiterWithOutPut (SubVI).vi"("VISA Refnum in"=w1239) -> ("Boolean"=w1237:bool)  [unwired: 10 in]
                                }
                              }
                              frame #5 {
                                # "Keeps the AMF valve after column-1 open and valve after column-2 closed"
                                n781 = local read "Buffer-C1 Dispense\nFlow Rate (ul/min) \nfor Equilibration\nof Column-2"() -> (w1253:dbl)
                                n782 = local read "Buffer-C1 Pumping\nResolution \nfor Equilibration \nof Column-2"() -> (w1252:T2)
                                n783 = local read "VISA Refnum in\nfor Pump"() -> (w1255:refnum<visa-resource-name>)
                                n784 = local write "Pause Data Collection"(FALSE ("Pause Data Collection")) -> ()
                                n785 = local read "Volume of Syringe"() -> (w1254:dbl)
                                n786 = call "GoToAbsolutePosition(SubVI).vi"("Absolute Volume Position in Syringe (in ul)"=0.0, "Volume of Syringe"=w1254, "Resolution of Pumping"=w1252, "Flow Rate (ul/min)"=w1253, "VISA Refnum in"=w1255) -> ()  [unwired: 6 in, 1 out]
                                n787 = local read "VISA Refnum in\nfor Valve"() -> (w1245:refnum<visa-resource-name>)
                                n788 = local write "Valve V1 Open"(FALSE ("Valve V1 Open")) -> ()
                                n789 = local write "Valve V2 Open"(TRUE ("Valve V2 Open")) -> ()
                                n790 = local write "Valve V3 Open"(TRUE ("Valve V3 Open")) -> ()
                                n791 = local write "Valve V4 Open"(FALSE ("Affinity On")) -> ()
                                n792 = local read "External Valve \nOPEN"() -> (w1244:string)
                                n793 = local write "Valve V5 Open"(FALSE ("Valve V5 Open")) -> ()
                                n794 = local write "Valve V6 Open"(FALSE ("Valve V6 Open")) -> ()
                                n795 = local write "Valve V7 Open"(FALSE ("Valve V7 Open")) -> ()
                                n796 = call "PortChanger_Valve (SubVI).vi"("Port Number"=w1244, "VISA Refnum in"=w1245) -> ()  [unwired: 10 in]
                              }
                              frame #6 {
                                n797 = local read "Buffer-C1 Pumping\nResolution \nfor Equilibration \nof Column-2"() -> (w1257:T2)
                                n798 = local read "VISA Refnum in\nfor Pump"() -> (w1259:refnum<visa-resource-name>)
                                n799 = local read "Initial Plunger Position"() -> (w1258:dbl)
                                n800 = local read "Volume of Syringe"() -> (w1256:dbl)
                                n801 = while {
                                tunnel: w1258 -> [w1266]
                                tunnel: w1259 -> [w1265]
                                tunnel: w1257 -> [w1264]
                                tunnel: w1256 -> [w1263]
                                stop <- w1261 stop-if-true
                                n802 = stacked-sequence {
                                tunnel: w1266 -> [w1273 _]
                                tunnel: w1265 -> [w1272 w1297]
                                tunnel: w1264 -> [w1271 _]
                                tunnel: w1263 -> [w1270 _]
                                tunnel: [_ w1295] -> w1261
                                frame #0 {
                                n803 = call "AbsolutePlungerPosition (SubVI).vi"("VISA Refnum in"=w1272) -> ("Plunger Position"=w1269:i32)  [unwired: 10 in]
                                n804 = case shown="\"Standard Pumping\", Default" w1271 {
                                tunnel: w1273 -> [w1278 w1287]
                                tunnel: w1269 -> [w1279 w1286]
                                tunnel: [w1277 w1284] -> w1268
                                tunnel: w1270 -> [w1276 w1285]
                                frame "Standard Pumping", Default {
                                n805 = Subtract(x=w1278, y=w1279) -> (x-y=w1275:dbl)
                                n806 = Absolute Value(x=w1275) -> (abs(x)=w1274:dbl)
                                n807 = Multiply(x=w1274, y=w1276) -> (x*y=w1281:dbl)
                                n808 = Divide(x=w1281, y=3000.0) -> (x/y=w1277:dbl)
                                }
                                frame "High Resolution Pumping" {
                                n809 = Subtract(x=w1287, y=w1286) -> (x-y=w1283:dbl)
                                n810 = Absolute Value(x=w1283) -> (abs(x)=w1282:dbl)
                                n811 = Multiply(x=w1282, y=w1285) -> (x*y=w1289:dbl)
                                n812 = Divide(x=w1289, y=24000.0) -> (x/y=w1284:dbl)
                                }
                                }
                                n813 = local write "Volume being Injected \nin this process"(w1268) -> ()
                                }
                                frame #1 {
                                n814 = local read "Buffer-C Volume \nto be Pumped for\nColumn \nnon-interference"() -> (w1293:dbl)
                                n815 = local read "Volume being Injected \nin this process"() -> (w1294:dbl)
                                n816 = local read "Stopper that ends \nthe main loops"() -> (w1292:bool)
                                n817 = call "LSPOneStatus (SubVI).vi"("VISA Refnum in"=w1297) -> ("read buffer"=w1299:string)  [unwired: 10 in]
                                n818 = call <vilib>:"Trim Whitespace.vi"("string"=w1299) -> ("trimmed string"=w1298:string)  [unwired: 1 in]
                                n819 = Equal?(x=w1298, y="/0`\u0003") -> (x = y?=w1296:bool)
                                n820 = Greater Or Equal?(x=w1294, y=w1293) -> (x >= y?=w1291:bool)
                                n821 = Or(x=w1292, y=w1291) -> (x .or. y?=w1290:bool)
                                n822 = Or(x=w1296, y=w1290) -> (x .or. y?=w1295:bool)
                                }
                                }
                                n823 = Wait (ms)(milliseconds to wait=u32 100) -> ()  [unwired: 1 out]
                                n824 = local read "Stopper that ends \nthe main loops"() -> (w1260:bool)
                                n825 = case shown="True" w1260 {
                                frame False {
                                }
                                frame True {
                                n826 = local read "VISA Refnum in\nfor Pump"() -> (w1267:refnum<visa-resource-name>)
                                n827 = call "HardStopCurrentProcess (SubVI).vi"("VISA Refnum in"=w1267) -> ()  [unwired: 11 in]
                                }
                                }
                                }
                              }
                              frame #7 {
                                # "Keeps the AMF valve after column-1 closed and valve after column-2 open"
                                n828 = local read "VISA Refnum in\nfor Valve"() -> (w1305:refnum<visa-resource-name>)
                                n829 = local read "External Valve \nCLOSED"() -> (w1304:string)
                                n830 = local write "Valve V4 Open"(TRUE ("Valve V4 Open")) -> ()
                                n831 = local write "Valve V1 Open"(FALSE ("Valve V1 Open")) -> ()
                                n832 = local write "Valve V2 Open"(FALSE ("Valve V2 Open")) -> ()
                                n833 = local write "Valve V3 Open"(FALSE ("Valve V3 Open")) -> ()
                                n834 = call "PortChanger_Valve (SubVI).vi"("Port Number"=w1304, "VISA Refnum in"=w1305) -> ()  [unwired: 10 in]
                                n835 = local write "Valve V7 Open"(TRUE ("Valve V7 Open")) -> ()
                                n836 = local write "Valve V5 Open"(TRUE ("Valve V5 Open")) -> ()
                                n837 = local write "Valve V6 Open"(TRUE ("Valve V6 Open")) -> ()
                              }
                              frame #8 {
                                n838 = local read "Buffer-C1 Pumping\nResolution \nfor Equilibration \nof Column-2"() -> (w1311:T2)
                                n839 = local read "VISA Refnum in\nfor Pump"() -> (w1313:refnum<visa-resource-name>)
                                n840 = local read "Initial Plunger Position"() -> (w1312:dbl)
                                n841 = local read "Volume of Syringe"() -> (w1310:dbl)
                                n842 = while {
                                tunnel: w1312 -> [w1320]
                                tunnel: w1313 -> [w1319]
                                tunnel: w1311 -> [w1318]
                                tunnel: w1310 -> [w1317]
                                stop <- w1315 stop-if-true
                                n843 = stacked-sequence {
                                tunnel: w1320 -> [w1327 _]
                                tunnel: w1319 -> [w1326 w1347]
                                tunnel: w1318 -> [w1325 _]
                                tunnel: w1317 -> [w1324 _]
                                tunnel: [_ w1345] -> w1315
                                frame #0 {
                                n844 = call "AbsolutePlungerPosition (SubVI).vi"("VISA Refnum in"=w1326) -> ("Plunger Position"=w1323:i32)  [unwired: 10 in]
                                n845 = case shown="\"Standard Pumping\", Default" w1325 {
                                tunnel: w1327 -> [w1332 w1341]
                                tunnel: w1323 -> [w1333 w1340]
                                tunnel: [w1331 w1338] -> w1322
                                tunnel: w1324 -> [w1330 w1339]
                                frame "Standard Pumping", Default {
                                n846 = Subtract(x=w1332, y=w1333) -> (x-y=w1329:dbl)
                                n847 = Absolute Value(x=w1329) -> (abs(x)=w1328:dbl)
                                n848 = Multiply(x=w1328, y=w1330) -> (x*y=w1335:dbl)
                                n849 = Divide(x=w1335, y=3000.0) -> (x/y=w1331:dbl)
                                }
                                frame "High Resolution Pumping" {
                                n850 = Subtract(x=w1341, y=w1340) -> (x-y=w1337:dbl)
                                n851 = Absolute Value(x=w1337) -> (abs(x)=w1336:dbl)
                                n852 = Multiply(x=w1336, y=w1339) -> (x*y=w1343:dbl)
                                n853 = Divide(x=w1343, y=24000.0) -> (x/y=w1338:dbl)
                                }
                                }
                                n854 = local write "Volume being Injected \nin this process"(w1322) -> ()
                                }
                                frame #1 {
                                n855 = local read "Stopper that ends \nthe main loops"() -> (w1344:bool)
                                n856 = call "LSPOneStatus (SubVI).vi"("VISA Refnum in"=w1347) -> ("read buffer"=w1349:string)  [unwired: 10 in]
                                n857 = call <vilib>:"Trim Whitespace.vi"("string"=w1349) -> ("trimmed string"=w1348:string)  [unwired: 1 in]
                                n858 = Equal?(x=w1348, y="/0`\u0003") -> (x = y?=w1346:bool)
                                n859 = Or(x=w1346, y=w1344) -> (x .or. y?=w1345:bool)
                                }
                                }
                                n860 = Wait (ms)(milliseconds to wait=u32 100) -> ()  [unwired: 1 out]
                                n861 = local read "Stopper that ends \nthe main loops"() -> (w1314:bool)
                                n862 = case shown="True" w1314 {
                                frame False {
                                }
                                frame True {
                                n863 = local read "VISA Refnum in\nfor Pump"() -> (w1321:refnum<visa-resource-name>)
                                n864 = call "HardStopCurrentProcess (SubVI).vi"("VISA Refnum in"=w1321) -> ()  [unwired: 11 in]
                                }
                                }
                                }
                              }
                              frame #9 {
                                n865 = local write "Pause Data Collection"(TRUE ("Pause Data Collection")) -> ()
                                n866 = Wait (ms)(milliseconds to wait=u32 500) -> ()  [unwired: 1 out]
                              }
                              frame #10 {
                                n867 = local write "Volume being Injected \nin this process"(0.0 ("Volume being Injected \nin this process")) -> ()
                                n868 = local write "Start the Process"(FALSE ("Start the Process")) -> ()
                              }
                            }
                          }
                          frame #10 {
                            # "Clean the tubing with Sample"
                            n869 = local read "N-S"() -> (w1355:i32)
                            n870 = for {
                              N: w1355 -> [_]
                              n871 = stacked-sequence {
                                frame #0 {
                                n872 = local read "VISA Refnum in\nfor Pump"() -> (w1358:refnum<visa-resource-name>)
                                n873 = local read "Port for \nSample"() -> (w1357:string)
                                n874 = call "PortChanger (SubVI).vi"("Port Number"=w1357, "VISA Refnum in"=w1358) -> ()  [unwired: 10 in]
                                }
                                frame #1 {
                                n875 = local read "VISA Refnum in\nfor Pump"() -> (w1359:refnum<visa-resource-name>)
                                n876 = call "ProcessCompletionWaiter (SubVI).vi"("VISA Refnum in"=w1359) -> ()  [unwired: 11 in]
                                }
                                frame #2 {
                                n877 = local read "VISA Refnum in\nfor Pump"() -> (w1364:refnum<visa-resource-name>)
                                n878 = local read "Sample PickUp \nFlow Rate (ul/min)"() -> (w1361:dbl)
                                n879 = local read "V-S"() -> (w1360:dbl)
                                n880 = local read "Volume of Syringe"() -> (w1362:dbl)
                                n881 = call "RPickUp(SubVI).vi"("Volume to be picked up"=w1360, "Volume of Syringe"=w1362, "Resolution of PickUP"=T2."Standard Pumping", "PickUp Flow Rate (ul/min)"=w1361, "VISA Refnum in"=w1364) -> ()  [unwired: 6 in, 1 out]
                                }
                                frame #3 {
                                n882 = local read "Stopper that ends \nthe main loops"() -> (w1365:bool)
                                n883 = local read "VISA Refnum in\nfor Pump"() -> (w1366:refnum<visa-resource-name>)
                                n884 = case shown="True" w1365 {
                                frame False {
                                }
                                frame True {
                                n885 = local read "VISA Refnum in\nfor Pump"() -> (w1367:refnum<visa-resource-name>)
                                n886 = call "HardStopCurrentProcess (SubVI).vi"("VISA Refnum in"=w1367) -> ()  [unwired: 11 in]
                                }
                                }
                                n887 = call "ProcessCompletionWaiter (SubVI).vi"("VISA Refnum in"=w1366) -> ()  [unwired: 11 in]
                                }
                                frame #4 {
                                n888 = local read "VISA Refnum in\nfor Pump"() -> (w1369:refnum<visa-resource-name>)
                                n889 = call "PortChanger (SubVI).vi"("Port Number"="1", "VISA Refnum in"=w1369) -> ()  [unwired: 10 in]
                                }
                                frame #5 {
                                n890 = local read "Stopper that ends \nthe main loops"() -> (w1370:bool)
                                n891 = local read "VISA Refnum in\nfor Pump"() -> (w1371:refnum<visa-resource-name>)
                                n892 = case shown="True" w1370 {
                                frame False {
                                }
                                frame True {
                                n893 = local read "VISA Refnum in\nfor Pump"() -> (w1372:refnum<visa-resource-name>)
                                n894 = call "HardStopCurrentProcess (SubVI).vi"("VISA Refnum in"=w1372) -> ()  [unwired: 11 in]
                                }
                                }
                                n895 = call "ProcessCompletionWaiter (SubVI).vi"("VISA Refnum in"=w1371) -> ()  [unwired: 11 in]
                                }
                                frame #6 {
                                n896 = local read "VISA Refnum in\nfor Pump"() -> (w1377:refnum<visa-resource-name>)
                                n897 = local read "Volume of Syringe"() -> (w1374:dbl)
                                n898 = call "GoToAbsolutePosition(SubVI).vi"("Absolute Volume Position in Syringe (in ul)"=0.0 ("Volume to be picked up"), "Volume of Syringe"=w1374, "Resolution of Pumping"=T2."Standard Pumping" ("Resolution of PickUP"), "Flow Rate (ul/min)"=150.0 ("PickUp Flow Rate (ul/min)"), "VISA Refnum in"=w1377) -> ()  [unwired: 6 in, 1 out]
                                }
                                frame #7 {
                                n899 = local read "Stopper that ends \nthe main loops"() -> (w1378:bool)
                                n900 = local read "VISA Refnum in\nfor Pump"() -> (w1379:refnum<visa-resource-name>)
                                n901 = case shown="True" w1378 {
                                frame False {
                                }
                                frame True {
                                n902 = local read "VISA Refnum in\nfor Pump"() -> (w1380:refnum<visa-resource-name>)
                                n903 = call "HardStopCurrentProcess (SubVI).vi"("VISA Refnum in"=w1380) -> ()  [unwired: 11 in]
                                }
                                }
                                n904 = call "ProcessCompletionWaiter (SubVI).vi"("VISA Refnum in"=w1379) -> ()  [unwired: 11 in]
                                }
                              }
                              n905 = local write "Pause Data Collection"(TRUE ("Pause Data Collection")) -> ()
                            }
                          }
                        }
                        n906 = local write "Equilibriating \nColumn-1"(TRUE ("Equilibriating \nColumn-1")) -> ()
                      }
                      frame #1 {
                        # "Pump Sample into Column-1"
                        n907 = stacked-sequence {
                          frame #0 {
                            # "Switch to Port-3"
                            # "Port-3 of pump is connected to Sample"
                            n908 = local read "VISA Refnum in\nfor Pump"() -> (w1385:refnum<visa-resource-name>)
                            n909 = local read "Port for \nSample"() -> (w1384:string)
                            n910 = call "PortChanger (SubVI).vi"("Port Number"=w1384, "VISA Refnum in"=w1385) -> ()  [unwired: 10 in]
                          }
                          frame #1 {
                            n911 = local read "VISA Refnum in\nfor Pump"() -> (w1386:refnum<visa-resource-name>)
                            n912 = call "ProcessCompletionWaiter (SubVI).vi"("VISA Refnum in"=w1386) -> ()  [unwired: 11 in]
                          }
                          frame #2 {
                            # "V4 is open"
                            # "V1, V2 and V3 are closed"
                            n913 = local read "VISA Refnum in\nfor Valve"() -> (w1391:refnum<visa-resource-name>)
                            n914 = local read "External Valve \nOPEN"() -> (w1390:string)
                            n915 = local write "Valve V1 Open"(TRUE ("Valve V1 Open")) -> ()
                            n916 = local write "Valve V2 Open"(TRUE ("Valve V2 Open")) -> ()
                            n917 = local write "Valve V3 Open"(FALSE ("Valve V3 Open")) -> ()
                            n918 = local write "Valve V4 Open"(FALSE ("Valve V4 Open")) -> ()
                            n919 = call "PortChanger_Valve (SubVI).vi"("Port Number"=w1390, "VISA Refnum in"=w1391) -> ()  [unwired: 10 in]
                            n920 = local write "Valve V5 Open"(FALSE ("Valve V5 Open")) -> ()
